vi "Spartan HTTP Verify Absolute Path.vi"(8 "reply in":T2, 9 "request":string="/c/web/home sweet home/access/internals/", 10 "absolute path":string="/c/web/home sweet home/access/internals/", 11 "env":T1) -> (0 "reply":T2, 1 "document path":string, 2 "document directory path":string, 3 "env out":T1, 4 "failed":bool)   [LabVIEW 2011]
uses:
  Addons/internet/http/cgi.llb/CGI Reply.ctl
  Addons/internet/utils/keyedarr.llb/Keyed Array.ctl
  OpenG.LIB/file/file.llb/Strip Path Extension - String__ogtk.vi
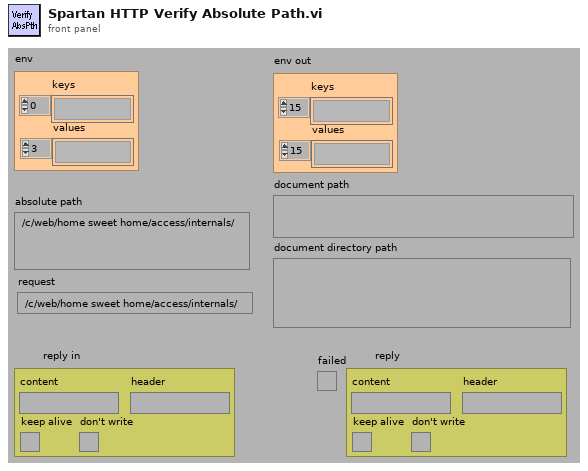
[diagram p1: front panel]
types:
  T1 = typedef "Keyed Array.ctl" = cluster{"keys":string[], "values":string[]}
  T2 = typedef "CGI Reply.ctl" = cluster{"content":string, "header":string, "keep alive":bool, "don't write":bool}
  T3 = enum32{"invalid app kind", "Development System", "Run Time System", "Student Edition", "Embedded LabVIEW", "Evaluation", "Custom"}
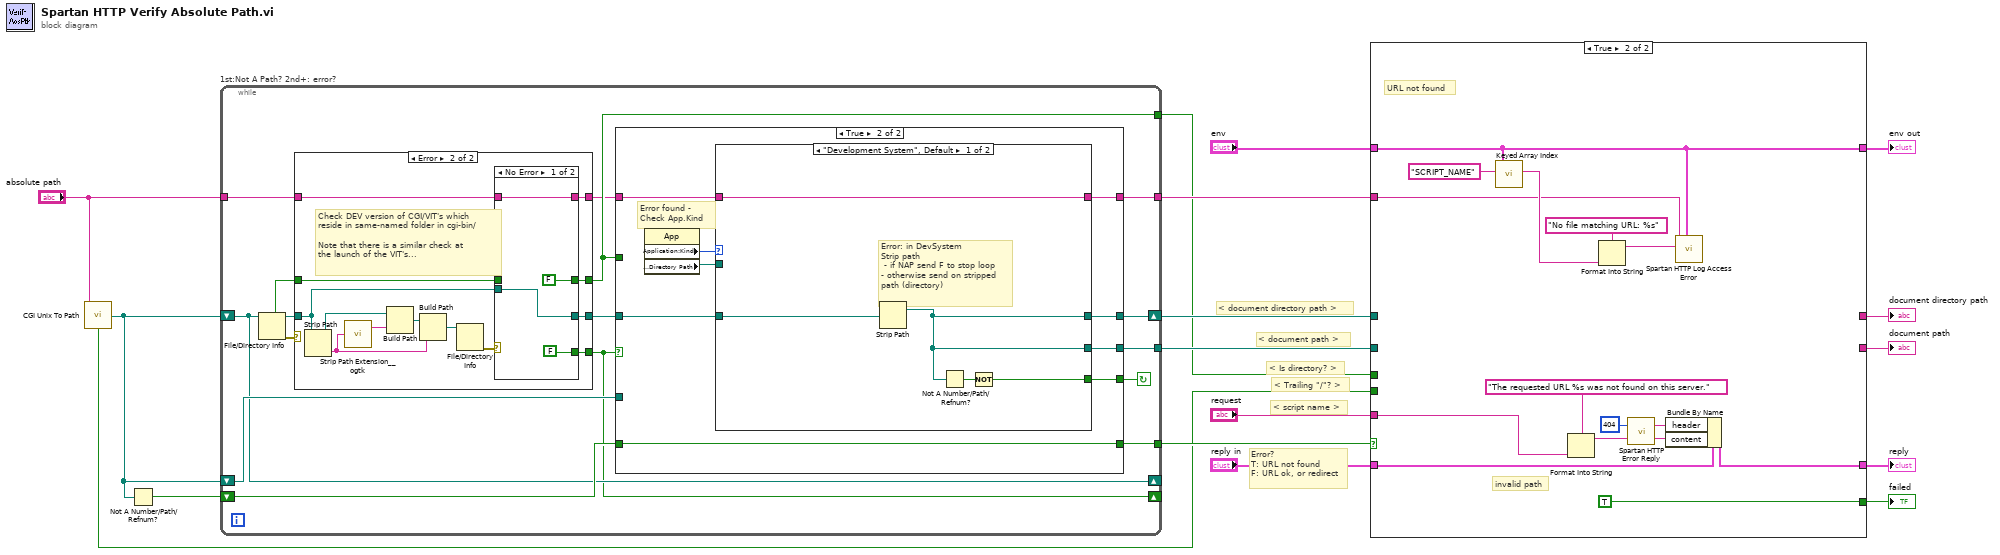
[diagram p0: block diagram]
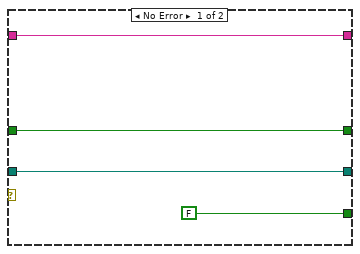
[diagram p2: hidden frame]
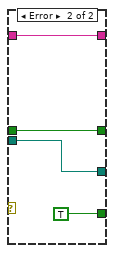
[diagram p3: hidden frame]
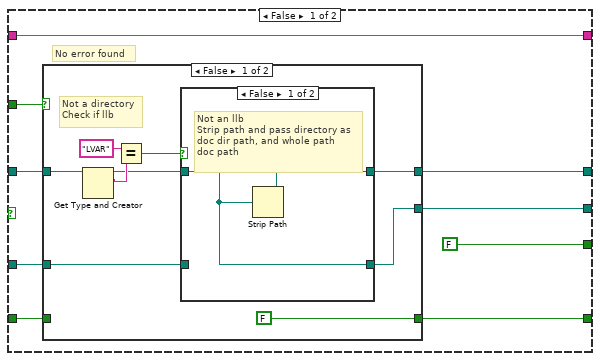
[diagram p4: hidden frame]
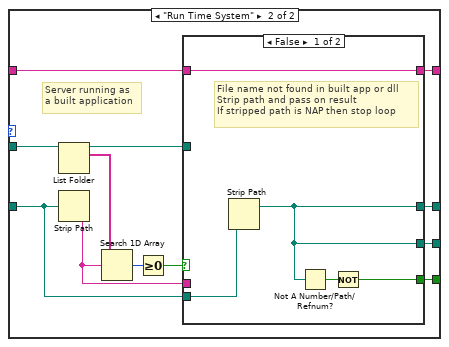
[diagram p7: hidden frame]
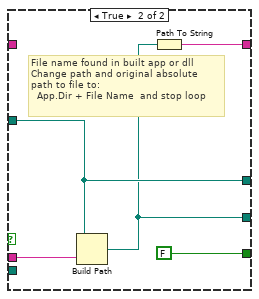
[diagram p8: hidden frame]
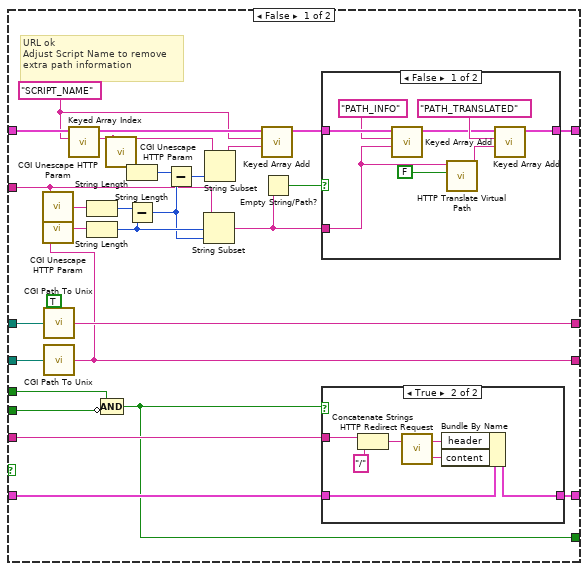
[diagram p9: hidden frame]
diagram:
  # "< Trailing \"/\"? >"
  # "< document directory path >"
  # "< document path >"
  # "Error?\nT: URL not found\nF: URL ok, or redirect"
  # "< Is directory? >"
  # "< script name >"
  n1 = call "CGI Unix To Path.vi"("unix path"="absolute path") -> ("trailing \"/\"?"=w5:bool, "platform path"=w14:path)
  n2 = Not A Number/Path/Refnum?(number/path/refnum=w14) -> (NaN/Path/Refnum?=w15:bool)
  n3 = while "1st:Not A Path? 2nd+: error?" {
    tunnel: [w20] -> w6
    tunnel: [w28] -> w11
    shift-left: w15 -> [w29]
    shift-right: [w22] -> _
    shift-left: w14 -> [w30]
    shift-right: [w27] -> _
    tunnel: [w31] -> w12
    shift-left: w14 -> [w27]
    shift-right: [w33] -> w13
    tunnel: "absolute path" -> [w19]
    tunnel: [w26] -> w9
    stop <- w32 continue-if-true
    n4 = File/Directory Info(path=w27) -> (path out=w24:path, directory=w21:bool, error out=w25:errorcluster)  [unwired: 1 in, 4 out]
    n5 = case shown="Error" w25 {
      tunnel: w24 -> [w37 w41]
      tunnel: [w37 w45] -> w23
      tunnel: [FALSE w43] -> w22
      tunnel: [w35 w44] -> w20
      tunnel: w21 -> [w35 w42]
      tunnel: w19 -> [w34 w40]
      tunnel: [w34 w39] -> w18
      frame No Error {
      }
      frame Error {
        # "Check DEV version of CGI/VIT's which\nreside in same-named folder in cgi-bin/\n\nNote that there is a similar check at\nthe launch of the VIT's..."
        n6 = Strip Path(path=w41) -> (stripped path=w48:path, name=w50:string)
        n7 = call-poly "Strip Path Extension__ogtk.vi"("path"=w50) -> ("root"=w38:string)  [unwired: 1 out]
        n8 = Build Path(base path=w48, name or relative path=w38) -> (appended path=w49:path)
        n9 = Build Path(base path=w49, name or relative path=w50) -> (appended path=w47:path)
        n10 = File/Directory Info(path=w47) -> (error out=w46:errorcluster)  [unwired: 1 in, 6 out]
        n11 = case shown="No Error" w46 {
          tunnel: [w51 w57] -> w45
          tunnel: [FALSE w58] -> w44
          tunnel: [FALSE TRUE] -> w43
          tunnel: w42 -> [_ w58]
          tunnel: w41 -> [w51 w57]
          tunnel: [w52 w55] -> w39
          tunnel: w40 -> [w52 w55]
          frame No Error {
          }
          frame Error {
          }
        }
      }
    }
    n12 = case shown="True" w22 {
      tunnel: w20 -> [w67 _]
      tunnel: w23 -> [w66 w91]
      tunnel: [w65 w87] -> w33
      tunnel: [FALSE w90] -> w32
      tunnel: [w63 w86] -> w31
      tunnel: w30 -> [w62 _]
      tunnel: w29 -> [w61 w89]
      tunnel: [w60 w89] -> w28
      tunnel: w18 -> [w59 w85]
      tunnel: [w59 w84] -> w26
      frame False {
        # "No error found"
        n13 = case shown="False" w67 {
          tunnel: w66 -> [w76 w82]
          tunnel: [w72 w82] -> w65
          tunnel: [w71 w82] -> w63
          tunnel: w62 -> [w70 _]
          tunnel: w61 -> [_ w81]
          tunnel: [FALSE ("status") w81] -> w60
          frame False {
            # "Not a directory\nCheck if llb"
            n14 = Get Type and Creator(7:w76) -> (2:w74:string, 3:w73:path)  [unwired: 1 in, 2 out]
            n15 = Equal?(x="LVAR", y=w74) -> (x = y?=w69:bool)
            n16 = case shown="False" w69 {
              tunnel: [w77 w79] -> w72
              tunnel: w73 -> [w78 w79]
              tunnel: [w78 w80] -> w71
              tunnel: w70 -> [_ w80]
              frame False {
                # "Not an llb\nStrip path and pass directory as\ndoc dir path, and whole path\ndoc path"
                n17 = Strip Path(path=w78) -> (stripped path=w77:path)  [unwired: 1 out]
              }
              frame True {
                # "It IS a llb\npass both paths unchanged"
              }
            }
          }
          frame True {
            # "It IS a directory"
          }
        }
      }
      frame True {
        # "Error found - \nCheck App.Kind"
        n18 = property class="App"() -> ("Application:Kind"=w88:T3, "Application:Directory Path"=w83:path)  [unwired: 2 in, 2 out]
        n19 = case shown="\"Development System\", Default" w88 {
          tunnel: w91 -> [w93 w98]
          tunnel: [w96 w105] -> w90
          tunnel: [w94 w107] -> w87
          tunnel: [w94 w106] -> w86
          tunnel: w85 -> [w95 w103]
          tunnel: [w95 w102] -> w84
          tunnel: w83 -> [_ w97]
          frame "Development System", Default {
            # "Error: in DevSystem\nStrip path\n - if NAP send F to stop loop\n- otherwise send on stripped\npath (directory)"
            n20 = Strip Path(path=w93) -> (stripped path=w94:path)  [unwired: 1 out]
            n21 = Not A Number/Path/Refnum?(number/path/refnum=w94) -> (NaN/Path/Refnum?=w92:bool)
            n22 = Not(x=w92) -> (.not. x?=w96:bool)
          }
          frame "Run Time System" {
            # "Server running as\na built application"
            n23 = List Folder(path=w97) -> (path out=w101:path, filenames=w104:string[])  [unwired: 1 in, 4 out]
            n24 = Strip Path(path=w98) -> (name=w99:string)  [unwired: 1 out]
            n25 = Search 1D Array(1D array=w104, element=w99) -> (index of element=w108:i32)  [unwired: 1 out]
            n26 = Greater Or Equal To 0?(x=w108) -> (x >= 0?=w100:bool)
            n27 = case shown="False" w100 {
              tunnel: w101 -> [_ w118]
              tunnel: [w112 w118] -> w107
              tunnel: [w112 w115] -> w106
              tunnel: [w110 FALSE] -> w105
              tunnel: w99 -> [_ w116]
              tunnel: w98 -> [w113 _]
              tunnel: w103 -> [w109 _]
              tunnel: [w109 w114] -> w102
              frame False {
                # "File name not found in built app or dll\nStrip path and pass on result\nIf stripped path is NAP then stop loop"
                n28 = Strip Path(path=w113) -> (stripped path=w112:path)  [unwired: 1 out]
                n29 = Not A Number/Path/Refnum?(number/path/refnum=w112) -> (NaN/Path/Refnum?=w111:bool)
                n30 = Not(x=w111) -> (.not. x?=w110:bool)
              }
              frame True {
                # "File name found in built app or dll\nChange path and original absolute\npath to file to:\n  App.Dir + File Name  and stop loop"
                n31 = Build Path(base path=w118, name or relative path=w116) -> (appended path=w115:path)
                n32 = Path To String(path=w115) -> (string=w114:string)
              }
            }
          }
        }
      }
    }
  }
  n33 = case shown="True" w11 {
    tunnel: w9 -> [w130 w175]
    tunnel: w12 -> [w147 _]
    tunnel: w13 -> [w146 _]
    tunnel: "env" -> [w141 w177]
    tunnel: [w143 w177] -> w16
    tunnel: [w131 _] -> w8
    tunnel: [w127 _] -> w7
    tunnel: w6 -> [w122 _]
    tunnel: w5 -> [w121 _]
    tunnel: "request" -> [w124 w166]
    tunnel: "reply in" -> [w123 w168]
    tunnel: [w120 TRUE] -> w2
    tunnel: [w119 w167] -> w1
    frame False {
      w139 = "SCRIPT_NAME" ("key")
      # "URL ok\nAdjust Script Name to remove\nextra path information"
      n34 = call "CGI Unescape HTTP Param.vi"("url-encoded string"=w130) -> ("string"=w129:string)
      n35 = call "CGI Path To Unix.vi"("platform path"=w146, "trailing \"/\"? (F)"=TRUE ("trailing \"/\"? (F)")) -> ("unix path"=w131:string)
      n36 = call "CGI Path To Unix.vi"("platform path"=w147) -> ("unix path"=w127:string)  [unwired: 1 in]
      n37 = call "CGI Unescape HTTP Param.vi"("url-encoded string"=w127) -> ("string"=w128:string)
      n38 = call "Keyed Array Index.vi"("key"=w139, "array in"=w141) -> ("value"=w126:string, "duplicate array"=w140:T1)  [unwired: 2 in, 2 out]
      n39 = String Length(string=w129) -> (length=w142:i32)
      n40 = String Length(string=w128) -> (length=w136:i32)
      n41 = Compound Arithmetic op=AND(w122, invert w121) -> (w120:bool)
      n42 = call "CGI Unescape HTTP Param.vi"("url-encoded string"=w126) -> ("string"=w125:string)
      n43 = String Length(string=w125) -> (length=w138:i32)
      n44 = Subtract(x=w142, y=w136) -> (x-y=w135:i32)
      n45 = Subtract(x=w138, y=w135) -> (x-y=w137:i32)
      n46 = String Subset(string=w130, offset (0)=w136, length (rest)=w135) -> (substring=w133:string)
      n47 = String Subset(string=w126, length (rest)=w137) -> (substring=w132:string)  [unwired: 1 out]
      n48 = call "Keyed Array Add.vi"("value"=w132, "key"=w139, "array in"=w140) -> ("array out"=w144:T1)  [unwired: 1 in, 3 out]
      n49 = Empty String/Path?(string/path=w133) -> (empty?=w134:bool)
      n50 = case shown="False" w134 {
        tunnel: w144 -> [w163 w164]
        tunnel: [w159 w164] -> w143
        tunnel: w133 -> [w156 _]
        frame False {
          n51 = call "Keyed Array Add.vi"("value"=w156, "key"="PATH_INFO", "array in"=w163) -> ("array out"=w160:T1)  [unwired: 1 in, 3 out]
          n52 = call "HTTP Translate Virtual Path.vi"("verify scope (T)"=FALSE, "virtual path"=w156) -> ("real path"=w158:string)  [unwired: 9 out]
          n53 = call "Keyed Array Add.vi"("value"=w158, "key"="PATH_TRANSLATED", "array in"=w160) -> ("array out"=w159:T1)  [unwired: 1 in, 3 out]
        }
        frame True {
        }
      }
      n54 = case shown="True" w120 {
        tunnel: [w148 w155] -> w119
        tunnel: w124 -> [_ w154]
        tunnel: w123 -> [w148 w153]
        frame False {
        }
        frame True {
          n55 = Concatenate Strings(w154, "/") -> (w152:string)
          n56 = call "HTTP Redirect Request.vi"("new location"=w152) -> ("content"=w150:string, "header"=w149:string)  [unwired: 1 out]
          n57 = Bundle By Name(cluster=w153, "header"=w149, "content"=w150) -> (w155:T2)
        }
      }
    }
    frame True {
      # "invalid path"
      # "URL not found"
      n58 = call "Keyed Array Index.vi"("key"="SCRIPT_NAME", "array in"=w177) -> ("value"=w176:string)  [unwired: 2 in, 3 out]
      n59 = Format Into String(format string="The requested URL %s was not found on this server.", w166) -> (resulting string=w173:string)  [unwired: 2 in, 1 out]
      n60 = Format Into String(format string="No file matching URL: %s", w176) -> (resulting string=w174:string)  [unwired: 2 in, 1 out]
      n61 = call "Spartan HTTP Error Reply.vi"("message"=w173, "status code"=404) -> ("content"=w170:string, "header"=w169:string)
      n62 = Bundle By Name(cluster=w168, "header"=w169, "content"=w170) -> (w167:T2)
      n63 = call "Spartan HTTP Log Access Error.vi"("env"=w177, "reason"=w174, "absolute path"=w175) -> ()  [unwired: 1 in, 8 out]
    }
  }
  "reply" <- w1
  "failed" <- w2
  "env out" <- w16
  "document directory path" <- w8
  "document path" <- w7
